vi "CreateUnsaturated.vi"(7 "unsat amount (2)":i32=2) -> (2 "Golden":refnum<queue>, 3 "POTTypedCircularBuffer out":refnum<class "POTTypedCircularBuffer.lvclass">)   [LabVIEW 2024, in "POTCircularBuffer.Tests.Units.lvlib"]
uses:
  POTCircularBuffer.Tests.Units.lvlib
  POTTypedCircularBuffer.lvclass
  Type.ctl
  POTTypedCircularBuffer.lvclass/POTTypedCircularBuffer.ctl
  Wrap.vi
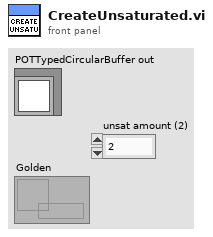
[diagram p1: front panel]
types:
  T1 = typedef "POTTypedCircularBuffer.lvclass/Type.ctl" = i32
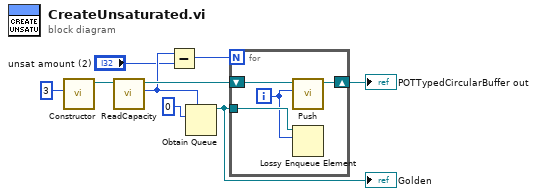
[diagram p0: block diagram]
diagram:
  n1 = call "Constructor.vi"("Capacity 2^n"=u32 3 ("Capacity")) -> ("POTTypedCircularBuffer out"=w8:refnum<class "POTTypedCircularBuffer.lvclass">)  [unwired: 10 in]
  n2 = call "ReadCapacity.vi"("POTTypedCircularBuffer in"=w8) -> ("capacity"=w3:i32, "POTTypedCircularBuffer out"=w7:refnum<class "POTTypedCircularBuffer.lvclass">)  [unwired: 9 in]
  n3 = Subtract(x=w3, y="unsat amount (2)") -> (x-y=w2:i32)
  n4 = Obtain Queue(max queue size (-1, unlimited)=w3, element data type=T1 0 ("Type")) -> (queue out=w4:refnum<queue>)  [unwired: 3 in, 2 out]
  "Golden" <- w4
  n5 = for {
    N: w2 -> [_]
    shift-right: [w12] -> w6
    shift-left: w7 -> [w13]
    tunnel: w4 -> [w11]
    i -> [w10]
    n6 = call "Push.vi"("Element"=w10, "POTTypedCircularBuffer in"=w13) -> ("POTTypedCircularBuffer out"=w12:refnum<class "POTTypedCircularBuffer.lvclass">)  [unwired: 9 in]
    n7 = Lossy Enqueue Element(queue=w11, element=w10) -> ()  [unwired: 1 in, 4 out]
  }
  "POTTypedCircularBuffer out" <- w6
